vi "ConvertValveList2CHFB.vi"() -> ()   [LabVIEW 2016]
panel:
  in  "Valve List":u16[](array[ring]) items=["A1", "A2", "A3", "A4", "B1", "B2", "B3", "B4", "B5", "B6", "B7", "B8", "A5"]
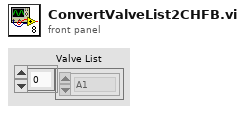
[diagram p1: front panel]
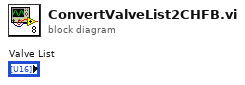
[diagram p0: block diagram]
diagram:
